vi "UDT_ErrorMonitorModule_ErrorPreRun.vi"() -> (3 "Unit Test Framework Results":T1)   [LabVIEW 2017]
doc: "Use this template to create a user-defined test VI. Define your test requirements and wire the results to the <b>Result (Test)</b> control. Do not modify the <b>Unit Test Framework Results</b> indicator."
uses:
  <vilib>/utf/common/utf_test_result_troll.ctl
  <vilib>/utf/common/utf_test_result.ctl
  <vilib>/utf/common/utf_test_result_failure.ctl
  <vilib>/utf/common/utf_test_comparison_operators.ctl
  <vilib>/utf/common/utf_vi_tag.ctl
  RT/ErrorMonitor/Queue/TypeDefs/queueFGVState.ctl
  RT/ErrorMonitor/Queue/TypeDefs/message.ctl
  <vilib>/Control Software Solutions Ltd/UTF Helper/SubVIs/UTF Variant Equals.vi
  <vilib>/Control Software Solutions Ltd/UTF Helper/Unit Test Helper.lvlib
  RT/ErrorMonitor/ErrorMonitor.lvlib
  <vilib>/utf/NI_UnitTestFramework.lvlib
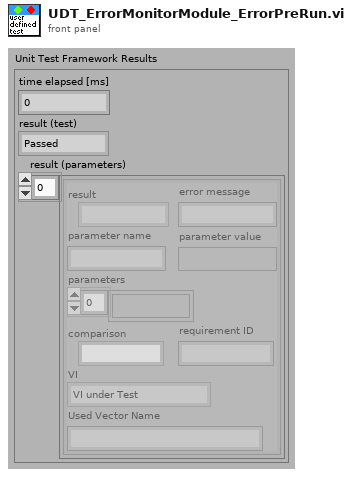
[diagram p1: front panel]
types:
  T1 = typedef "NI_UnitTestFramework.lvlib/utf_test_result_troll.ctl" = cluster{"time elapsed [ms]":u32, "result (test)":T2, "result (parameters)":T3[]}
  T2 = typedef "NI_UnitTestFramework.lvlib/utf_test_result.ctl" = enum16{"Passed", "Failed", "Error", "Skipped", "Not Processed"}
  T3 = typedef "NI_UnitTestFramework.lvlib/utf_test_result_failure.ctl" = cluster{"result":T2, "error message":string, "parameter name":string, "parameter value":variant, "parameters":variant[], "comparison":T4, "requirement ID":string, "VI":T5, "Used Vector Name":string}
  T4 = typedef "NI_UnitTestFramework.lvlib/utf_test_comparison_operators.ctl" = enum16{"=", "!=", ">", ">=", "<", "<=", "range", "symmetric tolerance", "asymmetric tolerance", "string contains", "string not contain", "array size", "string length", "array range", "by element", "array range (limit array)", "user-defined", "array contains", "array not contain", "vector length", "= (elm)", "!= (elm)", "= (case insensitive)", "!= (case insensitive)"}
  T5 = typedef "NI_UnitTestFramework.lvlib/utf_vi_tag.ctl" = enum16{"Setup VI", "VI under Test", "Teardown VI"}
  T6 = typedef "ErrorMonitor.lvlib/queueFGVState.ctl" = enum16{"obtain", "enqueue low priority", "enqueue high priority", "dequeue", "release"}
  T7 = typedef "ErrorMonitor.lvlib/message.ctl" = cluster{"calling module":string, "message":string, "Data":variant}
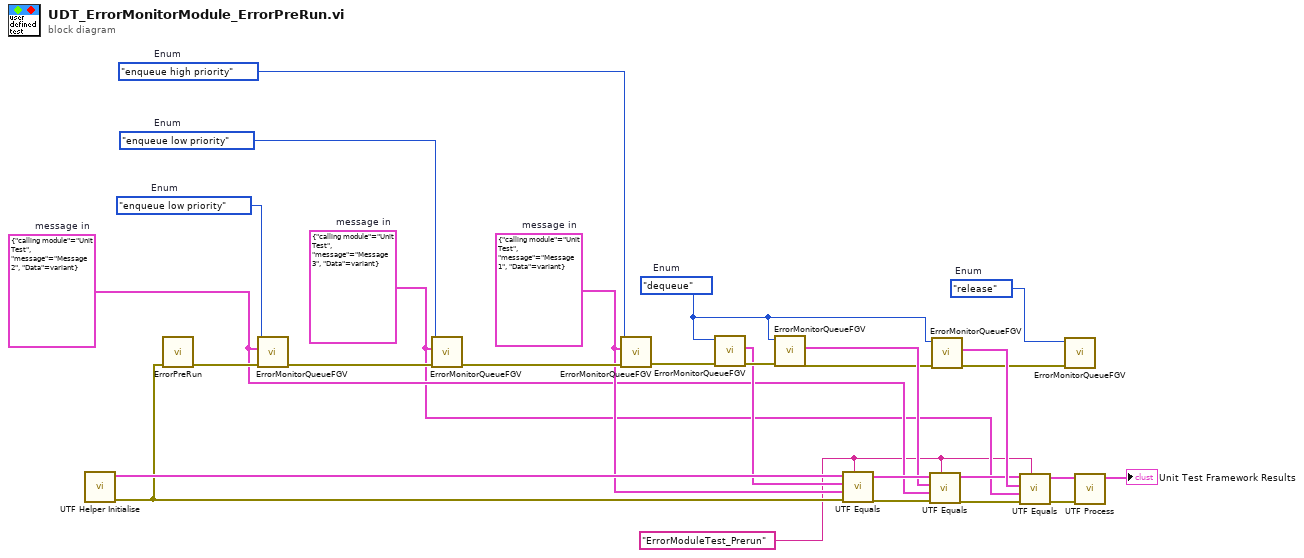
[diagram p0: block diagram]
diagram:
  w2 = "ErrorModuleTest_Prerun"
  w3 = queueFGVState."release"  # Enum
  w11 = queueFGVState."dequeue"  # Enum
  w20 = T7 {"calling module"="Unit Test", "message"="Message 1", "Data"=variant}  # message in
  w7 = T7 {"calling module"="Unit Test", "message"="Message 3", "Data"=variant}  # message in
  w13 = T7 {"calling module"="Unit Test", "message"="Message 2", "Data"=variant}  # message in
  w24 = queueFGVState."enqueue high priority"  # Enum
  w26 = queueFGVState."enqueue low priority"  # Enum
  w27 = queueFGVState."enqueue low priority"  # Enum
  n1 = call <vilib>:"UTF Helper Initialise.vi"() -> ("error out"=w21:errorcluster, "results array"=w22:T3[])  [unwired: 10 in]
  n2 = call "ErrorPreRun.vi"("error in (no error)"=w21) -> ("error out"=w28:errorcluster)  [unwired: 10 in]
  n3 = call "ErrorMonitorQueueFGV.vi"("error in (no error)"=w28, "message in"=w13, "Enum"=w27) -> ("error out"=w25:errorcluster)  [unwired: 7 in, 1 out]
  n4 = call "ErrorMonitorQueueFGV.vi"("error in (no error)"=w25, "message in"=w7, "Enum"=w26) -> ("error out"=w23:errorcluster)  [unwired: 7 in, 1 out]
  n5 = call "ErrorMonitorQueueFGV.vi"("error in (no error)"=w23, "message in"=w20, "Enum"=w24) -> ("error out"=w19:errorcluster)  [unwired: 7 in, 1 out]
  n6 = call "ErrorMonitorQueueFGV.vi"("error in (no error)"=w19, "Enum"=w11) -> ("error out"=w16:errorcluster, "message out"=w15:T7)  [unwired: 8 in]
  n7 = call "ErrorMonitorQueueFGV.vi"("error in (no error)"=w16, "Enum"=w11) -> ("error out"=w12:errorcluster, "message out"=w14:T7)  [unwired: 8 in]
  n8 = call-poly <vilib>:"UTF Equals.vi"("Parameter Name"=w2, "error in (no error)"=w21, "Test Value"=w20, "Input"=w15, "Input Results"=w22) -> ("error out"=w18:errorcluster, "Output Results"=w17:T3[])  [unwired: 5 in]
  n9 = call-poly <vilib>:"UTF Equals.vi"("Parameter Name"=w2, "error in (no error)"=w18, "Test Value"=w13, "Input"=w14, "Input Results"=w17) -> ("error out"=w8:errorcluster, "Output Results"=w9:T3[])  [unwired: 5 in]
  n10 = call "ErrorMonitorQueueFGV.vi"("error in (no error)"=w12, "Enum"=w11) -> ("error out"=w4:errorcluster, "message out"=w10:T7)  [unwired: 8 in]
  n11 = call-poly <vilib>:"UTF Equals.vi"("Parameter Name"=w2, "error in (no error)"=w8, "Test Value"=w7, "Input"=w10, "Input Results"=w9) -> ("error out"=w5:errorcluster, "Output Results"=w6:T3[])  [unwired: 5 in]
  n12 = call "ErrorMonitorQueueFGV.vi"("error in (no error)"=w4, "Enum"=w3) -> ()  [unwired: 8 in, 2 out]
  n13 = call <vilib>:"UTF Process.vi"("error in (no error)"=w5, "results array"=w6) -> ("Unit Test Framework Results"=→"Unit Test Framework Results":T1)  [unwired: 9 in]
